vi "Knob3.vi"(0 "PwrIn":dbl=10.0 format="%_7g", 2 "Knob":i8(knob)=1 scale=1.0..20.0, 3 "Step Size":dbl, 4 "Reset":bool, 5 "aup":bool, 6 "adn":bool) -> (8 "PwrSet":string="W1000.00", 10 "PwrOut":dbl)   [LabVIEW 2017]
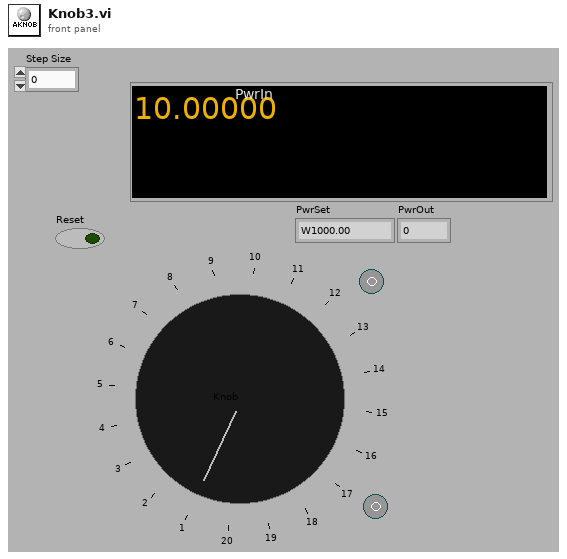
[diagram p1: front panel]
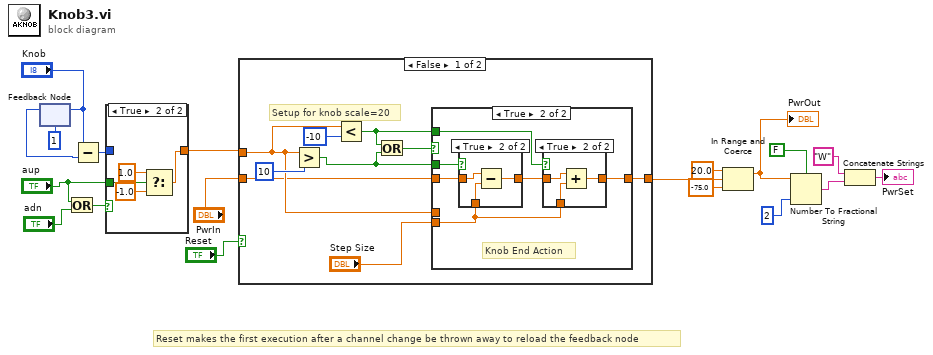
[diagram p0: block diagram]
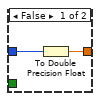
[diagram p2: hidden frame]
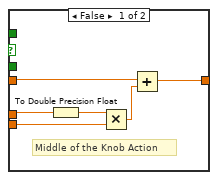
[diagram p3: hidden frame]
diagram:
  # "Reset makes the first execution after a channel change be thrown away to reload the feedback node"
  n1 = feedback-in #1("Knob") -> ()
  n2 = feedback #1(i8 1 ("Knob")) -> (w18:i8)
  n3 = Or(x="aup", y="adn") -> (x .or. y?=w14:bool)
  n4 = Subtract(x="Knob", y=w18) -> (x-y=w13:i8)
  n5 = case shown="True" w14 {
    tunnel: w13 -> [w20 _]
    tunnel: [w21 w24] -> w12
    tunnel: "aup" -> [_ w25]
    frame False {
      n6 = To Double Precision Float(number=w20) -> (double precision float=w21:dbl)
    }
    frame True {
      n7 = Select(t=1.0, s=w25, f=-1.0) -> (s? t:f=w24:dbl)
    }
  }
  n8 = case shown="False" "Reset" {
    tunnel: w12 -> [w29 _]
    tunnel: "PwrIn" -> [w28 w55]
    tunnel: [w27 w55] -> w4
    frame False {
      # "Setup for knob scale=20"
      n9 = Greater?(x=w29, y=10) -> (0:w31:bool)
      n10 = Less?(x=w29, y=-10) -> (x < y?=w30:bool)
      n11 = Or(x=w30, y=w31) -> (x .or. y?=w32:bool)
      n12 = case shown="True" w32 {
        tunnel: w31 -> [_ w46]
        tunnel: w28 -> [w39 w45]
        tunnel: w30 -> [_ w43]
        tunnel: [w40 w42] -> w27
        tunnel: "Step Size" -> [w38 w41]
        tunnel: w29 -> [w35 _]
        frame False {
          # "Middle of the Knob Action"
          n13 = To Double Precision Float(number=w35) -> (double precision float=w36:dbl)
          n14 = Multiply(x=w36, y=w38) -> (x*y=w37:dbl)
          n15 = Add(x=w39, y=w37) -> (x+y=w40:dbl)
        }
        frame True {
          # "Knob End Action"
          n16 = case shown="True" w46 {
            tunnel: w45 -> [w51 w53]
            tunnel: [w51 w54] -> w44
            tunnel: w41 -> [_ w52]
            frame False {
            }
            frame True {
              n17 = Subtract(x=w53, y=w52) -> (x-y=w54:dbl)
            }
          }
          n18 = case shown="True" w43 {
            tunnel: w44 -> [w47 w49]
            tunnel: [w47 w50] -> w42
            tunnel: w41 -> [_ w48]
            frame False {
            }
            frame True {
              n19 = Add(x=w49, y=w48) -> (x+y=w50:dbl)
            }
          }
        }
      }
    }
    frame True {
    }
  }
  n20 = In Range and Coerce(upper limit=20.0, x=w4, lower limit=-75.0) -> (coerced(x)=w3:dbl)  [unwired: 1 out]
  "PwrOut" <- w3
  n21 = Number To Fractional String(use system decimal point (T)=FALSE, number=w3, precision (6)=i16 2) -> (F-format string=w7:string)  [unwired: 1 in]
  n22 = Concatenate Strings("W" ("string"), w7) -> (→"PwrSet":string)
